vi "String_add_to_end.vi"(1 "Addition String":string, 2 "command line":string) -> (0 "result string":string)   [LabVIEW 2025]
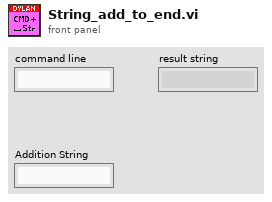
[diagram p1: front panel]
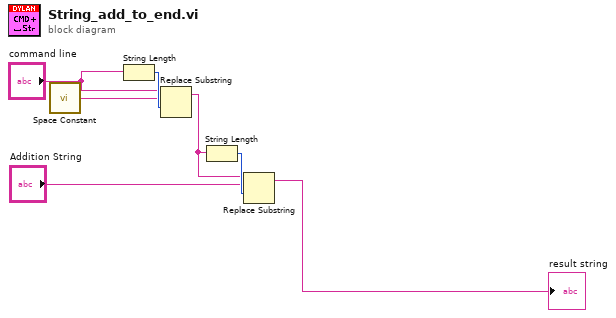
[diagram p0: block diagram]
diagram:
  n1 = call <vilib>:"Space Constant.vi"() -> ("String"=w3:string)
  n2 = String Length(string="command line") -> (length=w4:i32)
  n3 = Replace Substring(3:w4, 4:w3, 5:"command line") -> (1:w2:string)  [unwired: 1 in, 1 out]
  n4 = String Length(string=w2) -> (length=w6:i32)
  n5 = Replace Substring(3:w6, 4:"Addition String", 5:w2) -> (1:→"result string":string)  [unwired: 1 in, 1 out]
